vi "Test Coffee Shop Remove Cashier.vi"(8 "error in (no error)":errorcluster, 11 "Coffee Shop Test In":refnum<class "Coffee Shop Test.lvclass">) -> (0 "error out":errorcluster, 3 "Coffee Shop Test Out":refnum<class "Coffee Shop Test.lvclass">)   [LabVIEW 2020, in "Coffee Shop Test.lvclass"]
uses:
  Coffee Shop Test.lvclass
  Coffee Shop/Coffee Shop.lvclass
  <vilib>/Asteme/Triarc Framework/Process/Process.lvclass
  C:/Program Files (x86)/National Instruments/LabVIEW 2020/vi.lib/Asteme/Triarc Framework/Application/Application.lvclass
  C:/Program Files (x86)/National Instruments/LabVIEW 2020/vi.lib/Asteme/Triarc Framework/Process/Process.lvclass
  C:/Program Files (x86)/National Instruments/LabVIEW 2020/vi.lib/Asteme/Triarc Framework/Base/Base.lvclass
  C:/Program Files (x86)/National Instruments/LabVIEW 2020/vi.lib/Asteme/Triarc Framework/Error Handler Interface/Error Handler Interface.lvclass
  C:/Program Files (x86)/National Instruments/LabVIEW 2020/vi.lib/Asteme/Triarc Framework/Logging/Logging.lvclass
  C:/Users/anton/Documents/GitHub/Triarc-Examples/Coffee Shop/Coffee Shop/Coffee Shop.lvclass
  <vilib>/Asteme/Triarc Framework/Application/Application.lvclass
  <vilib>/Asteme/LUnit/Test Case.lvclass
  C:/Program Files (x86)/National Instruments/LabVIEW 2020/vi.lib/Asteme/Triarc Framework Test Suite/Application Test/Application Test.lvclass
  C:/Program Files (x86)/National Instruments/LabVIEW 2020/vi.lib/Asteme/Triarc Framework Test Suite/Process Test/Process Test.lvclass
  C:/Program Files (x86)/National Instruments/LabVIEW 2020/vi.lib/Asteme/Triarc Framework Test Suite/Base Class Test/Base Test.lvclass
  C:/Program Files (x86)/National Instruments/LabVIEW 2020/vi.lib/Asteme/LUnit/Test Case.lvclass
  C:/Users/anton/Documents/GitHub/Triarc-Examples/Coffee Shop/Coffee Shop Test/Coffee Shop Test.lvclass
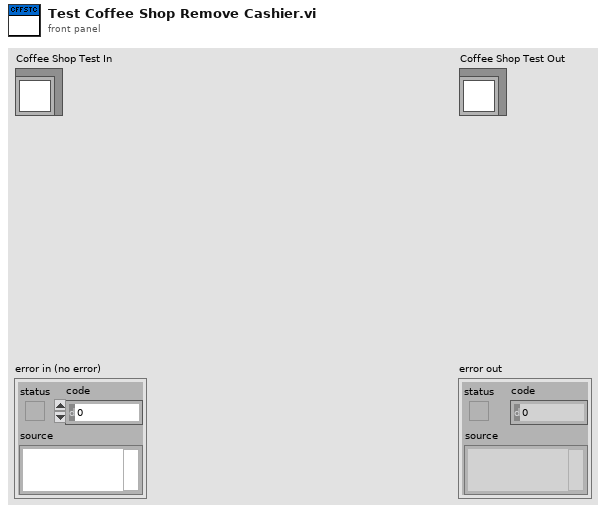
[diagram p1: front panel]
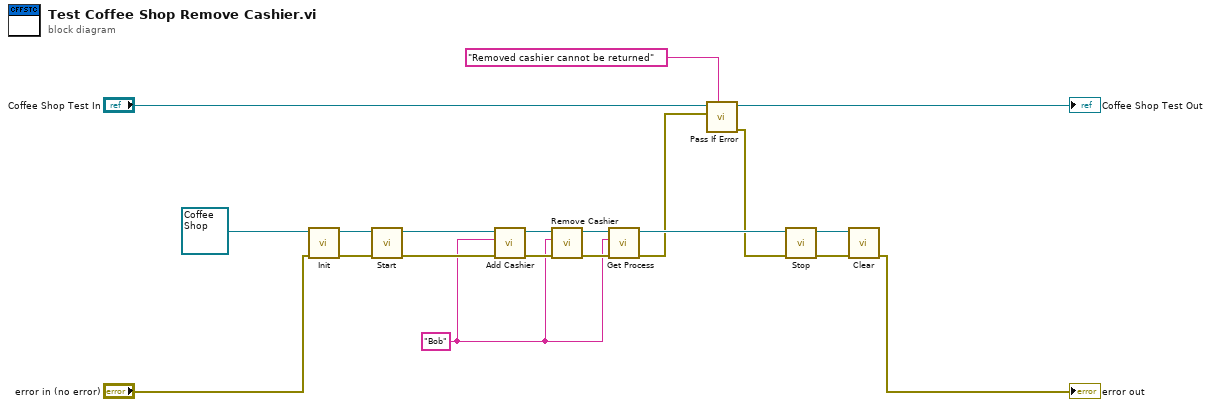
[diagram p0: block diagram]
diagram:
  w4 = "Bob" ("Name")
  n1 = call-dynamic "Init.vi"("error in (no error)"="error in (no error)", "Process In"=refnum<class "Coffee Shop.lvclass"> refnum ("Coffee Shop.lvclass")) -> ("error out"=w18:errorcluster, "Process Out"=w19:refnum<class "Coffee Shop.lvclass">)  [unwired: 8 in]
  n2 = call <vilib>:"Start.vi"("error in (no error)"=w18, "Process In"=w19) -> ("error out"=w13:errorcluster, "Process Out"=w12:refnum<class "Coffee Shop.lvclass">)  [unwired: 8 in]
  n3 = call "Add Cashier.vi"("error in (no error)"=w13, "Name"=w4, "Coffee Shop in"=w12) -> ("error out"=w14:errorcluster, "Coffee Shop out"=w6:refnum<class "Coffee Shop.lvclass">)  [unwired: 7 in]
  n4 = call "Remove Cashier.vi"("error in (no error)"=w14, "Name"=w4, "Coffee Shop In"=w6) -> ("error out"=w7:errorcluster, "Coffee Shop Out"=w5:refnum<class "Coffee Shop.lvclass">)  [unwired: 7 in]
  n5 = call <vilib>:"Get Process.vi"("error in (no error)"=w7, "Process Name"=w4, "Rig In"=w5) -> ("error out"=w3:errorcluster, "Rig Out"=w8:refnum<class "Coffee Shop.lvclass">)  [unwired: 6 in, 1 out]
  n6 = call <vilib>:"Pass If Error.vi"("Description"="Removed cashier cannot be returned", "Assert error"=w3, "Test Case In"="Coffee Shop Test In") -> ("error out"=w2:errorcluster, "Test Case Out"=→"Coffee Shop Test Out":refnum<class "Coffee Shop Test.lvclass">)  [unwired: 7 in]
  n7 = call <vilib>:"Stop.vi"("error in (no error)"=w2, "Process In"=w8) -> ("error out"=w16:errorcluster, "Process Out"=w17:refnum<class "Coffee Shop.lvclass">)  [unwired: 7 in, 1 out]
  n8 = call-dynamic "Clear.vi"("error in (no error)"=w16, "Application In"=w17) -> ("error out"=→"error out":errorcluster)  [unwired: 9 in]
